vi "DIMPowerSupply.ProcCases.vi"(0 "i ref in":refnum<vi>, 1 "selector":string, 2 "Data":T1, 3 "call cluster":T2={"Object"="", "Selector"="", "CallType"=enum."synchronous", "Async Object"="", "Async Selector"="", "Data Descriptor"="", "Data"=[], "Error #"=0, "Expire"=0}, 5 "error in (no error)":errorcluster) -> (14 "i ref out":refnum<vi>, 17 "answer cluster":T2={"Object"="", "Selector"="", "CallType"=enum."synchronous", "Async Object"="", "Async Selector"="", "Data Descriptor"="", "Data"=[], "Error #"=0, "Expire"=0}, 19 "error out":errorcluster)   [LabVIEW 2014, in "DIMPowerSupply.lvlib"]
doc: "This method is called by a process from within the default case in the event loop. The methods of a class that are linked to events will be called from THIS method. Add your code here."
uses:
  DIMPowerSupply.lvlib
  CS_Core/CSSystem/CoreDefs/CoreDefs.call_type.ctl
  CS_Core/BaseProcess/BaseProcess.descriptor string definition.ctl
  CS_Core/CSSystem/CoreDefs/CoreDefs.rawDataType.ctl
  CS_Core/CSSystem/CoreLib/CoreLib.byte array 2 double.vi
  CS_Core/CSSystem/CoreLib/CoreLib.string 2 byte array.vi
  CS_Core/CSSystem/CoreLib/CoreLib.byte array 2 int.vi
  CS_Core/BaseProcess/BaseProcess.lvlib
  CS_Core/CSSystem/CoreLib/CoreLib.lvlib
  CS_Core/CAEObj/CAEObj.lvlib
  CS_Core/CSApplicationBaseClasses/PSChannelBase/PSChannelBase.lvlib
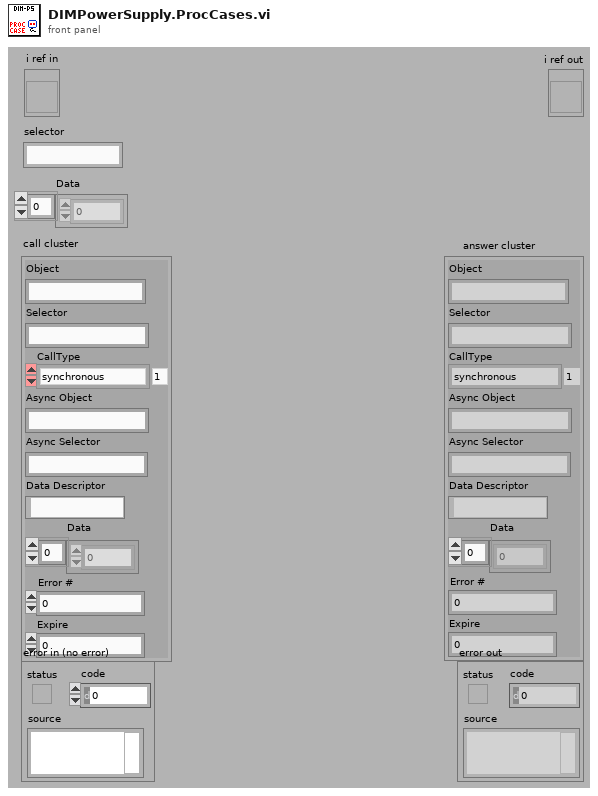
[diagram p1: front panel]
types:
  T1 = typedef "CoreDefs.rawDataType.ctl" = i8[]
  T2 = typedef "CoreDefs.call_type.ctl" = cluster{"Object":string, "Selector":string, "CallType":enum16{"simple", "synchronous", "asynchronous"}, "Async Object":string, "Async Selector":string, "Data Descriptor":T3, "Data":T1, "Error #":i32, "Expire":u32}
  T3 = typedef "BaseProcess.lvlib/BaseProcess.descriptor string definition.ctl" = string
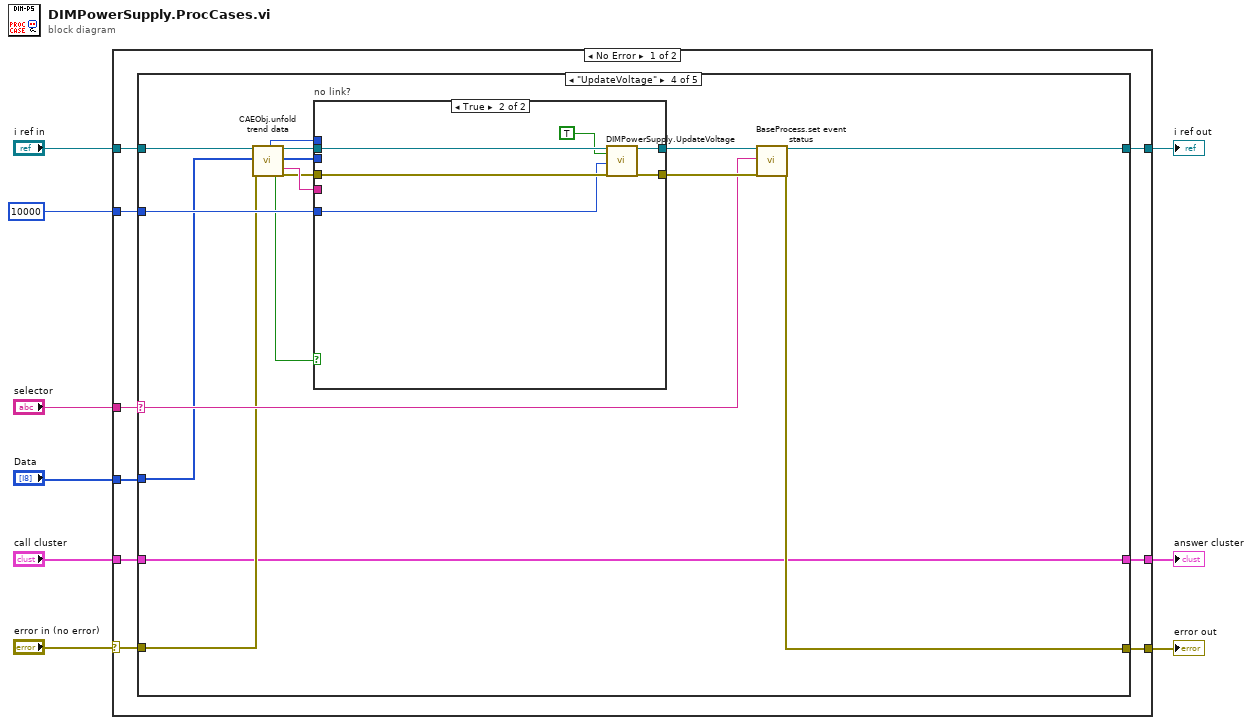
[diagram p0: block diagram]
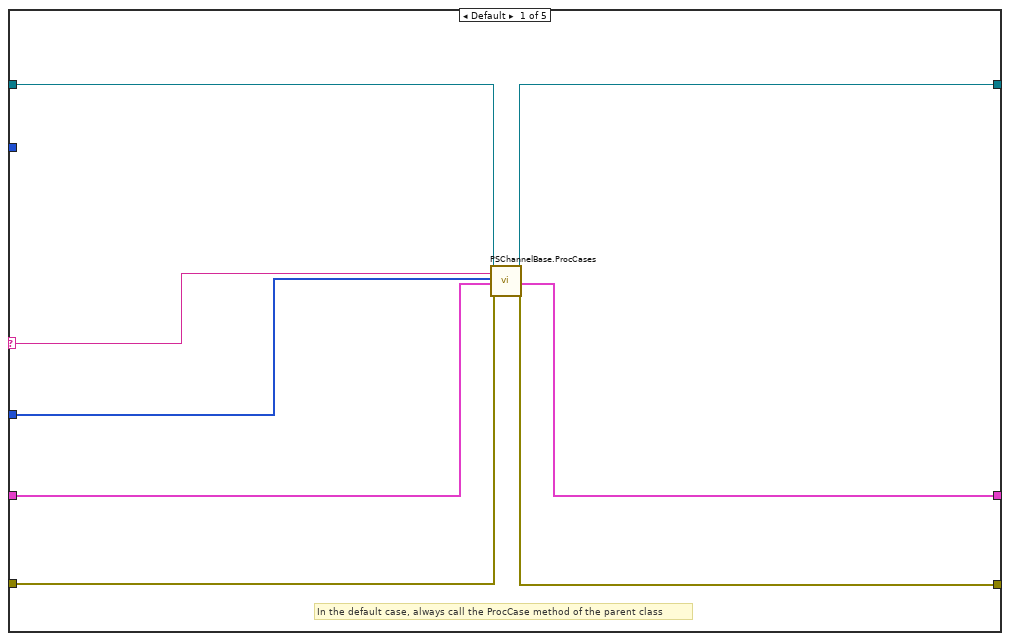
[diagram p2: hidden frame]
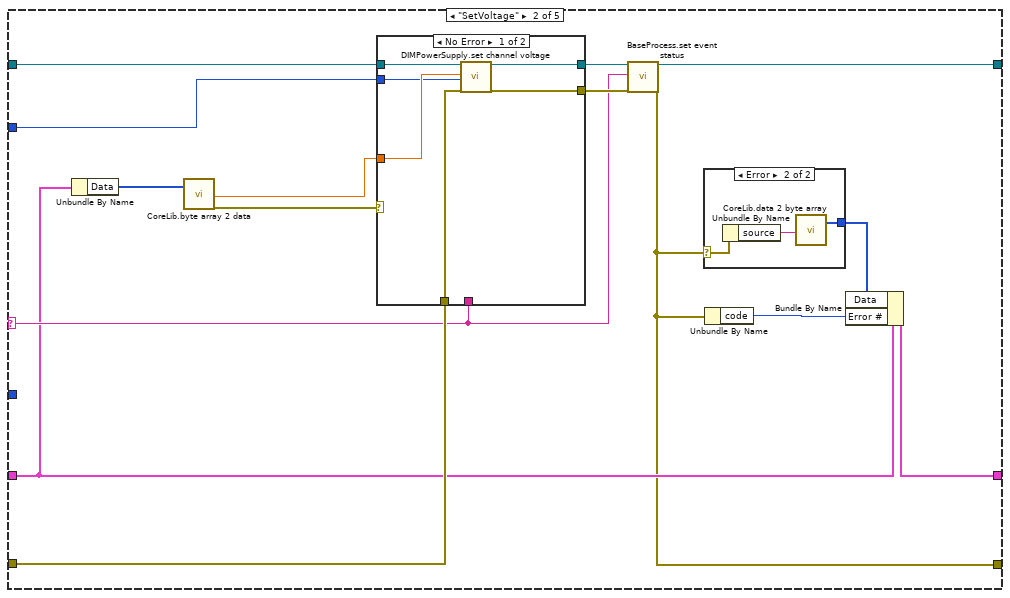
[diagram p3: hidden frame]
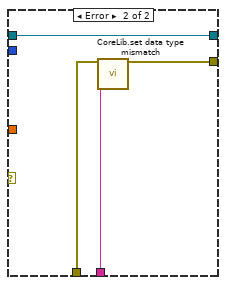
[diagram p4: hidden frame]
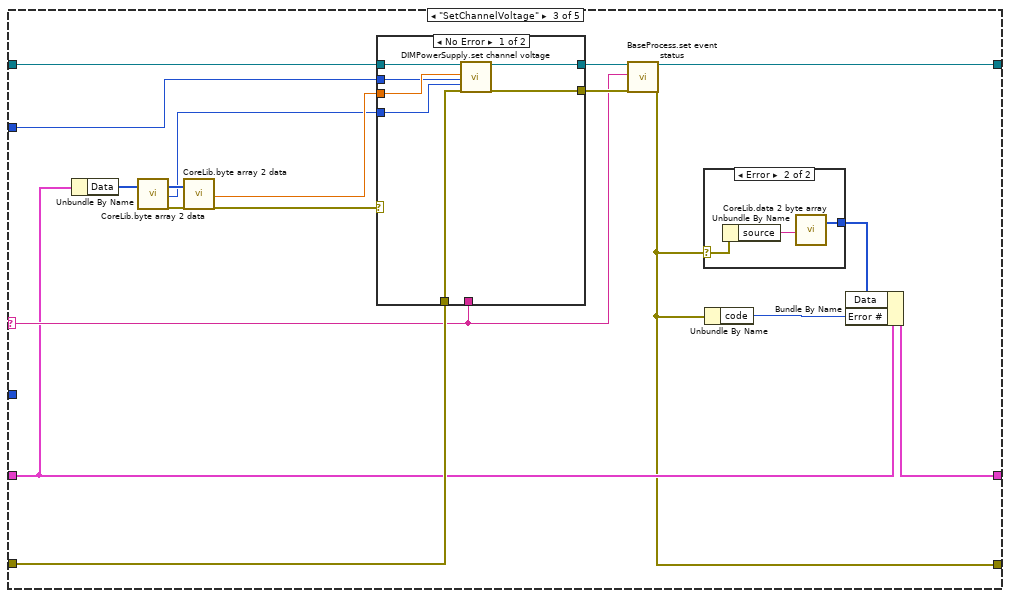
[diagram p6: hidden frame]
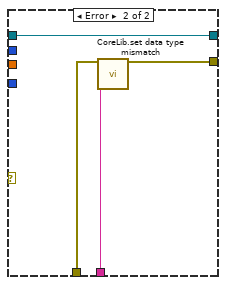
[diagram p7: hidden frame]
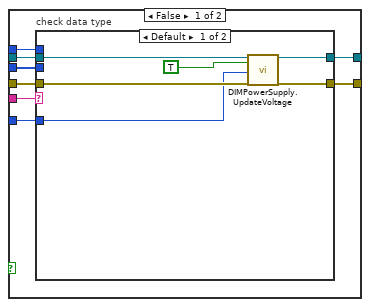
[diagram p9: hidden frame]
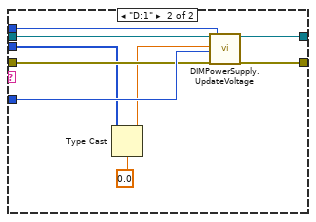
[diagram p10: hidden frame]
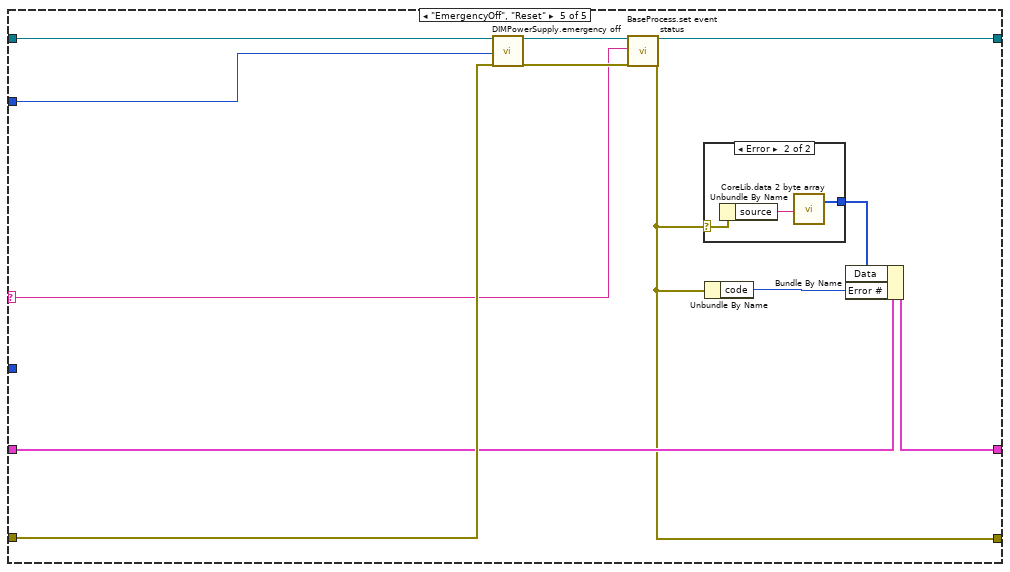
[diagram p11: hidden frame]
diagram:
  n1 = case shown="No Error" "error in (no error)" {
    selector: "error in (no error)" -> [w10 w147]
    tunnel: "selector" -> [w18 _]
    tunnel: [w17 w148] -> w8
    tunnel: "Data" -> [w16 _]
    tunnel: "call cluster" -> [w15 w148]
    tunnel: "i ref in" -> [w14 w149]
    tunnel: [w13 w149] -> w4
    tunnel: [w12 w147] -> w3
    tunnel: 10000 ("ms timeout (100)") -> [w11 _]
    frame No Error {
      n2 = case shown="\"UpdateVoltage\"" w18 {
        selector: w18 -> [w20 w35 w66 w100 w137]
        tunnel: w16 -> [w21 _ _ w96 _]
        tunnel: w14 -> [w19 w37 w68 w95 w139]
        tunnel: [w26 w30 w61 w97 w132] -> w13
        tunnel: w15 -> [w22 w33 w64 w88 w135]
        tunnel: [w23 w32 w63 w88 w134] -> w17
        tunnel: w10 -> [w25 w36 w67 w93 w138]
        tunnel: [w24 w31 w62 w98 w133] -> w12
        tunnel: w11 -> [_ w34 w65 w99 w136]
        frame Default {
          # "In the default case, always call the ProcCase method of the parent class"
          n3 = call "PSChannelBase.ProcCases.vi"("i ref in"=w19, "selector"=w20, "Data"=w21, "call cluster"=w22, "error in (no error)"=w25) -> ("i ref out"=w26:refnum<vi>, "answer cluster"=w23:T2, "error out"=w24:errorcluster)  [unwired: 12 in]
        }
        frame "SetVoltage" {
          n4 = Unbundle By Name(w33) -> ("Data"=w29:T1)
          n5 = call-poly "CoreLib.byte array 2 data.vi"("byteArray"=w29) -> ("d64"=w27:dbl, "error out"=w28:errorcluster)  [unwired: 16 in, 1 out]
          n6 = case shown="No Error" w28 {
            tunnel: [w47 w50] -> w40
            tunnel: [w46 w51] -> w41
            tunnel: w27 -> [w45 _]
            tunnel: w37 -> [w44 w50]
            tunnel: w36 -> [w43 w49]
            tunnel: w35 -> [_ w48]
            tunnel: w34 -> [w42 _]
            frame No Error {
              n7 = call "DIMPowerSupply.set channel voltage.vi"("i ref in"=w44, "Voltage"=w45, "ms timeout (10000)"=w42, "error in (no error)"=w43) -> ("i ref out"=w47:refnum<vi>, "error out"=w46:errorcluster)  [unwired: 13 in, 1 out]
            }
            frame Error {
              n8 = call "CoreLib.set data type mismatch.vi"("error in (no error)"=w49, "error source"=w48) -> ("error out"=w51:errorcluster)  [unwired: 17 in]
            }
          }
          n9 = call "BaseProcess.set event status.vi"("i ref in"=w40, "EventStatus"=w35, "error in (no error)"=w41) -> ("i ref out"=w30:refnum<vi>, "error out"=w31:errorcluster)  [unwired: 14 in, 1 out]
          n10 = case shown="Error" w31 {
            selector: w31 -> [_ w54]
            tunnel: [_ w52] -> w39
            frame No Error {
            }
            frame Error {
              n11 = Unbundle By Name(w54) -> ("source"=w53:string)
              n12 = call-poly "CoreLib.data 2 byte array.vi"("string"=w53) -> ("byteArray out"=w52:T1)  [unwired: 18 in]
            }
          }
          n13 = Unbundle By Name(w31) -> ("code"=w38:i32)
          n14 = Bundle By Name(cluster=w33, "Data"=w39, "Error #"=w38) -> (w32:T2)
        }
        frame "SetChannelVoltage" {
          n15 = Unbundle By Name(w64) -> ("Data"=w56:T1)
          n16 = call-poly "CoreLib.byte array 2 data.vi"("byteArray"=w56) -> ("byteArray out"=w58:T1, "i32"=w55:i32, "error out"=w57:errorcluster)  [unwired: 16 in]
          n17 = call-poly "CoreLib.byte array 2 data.vi"("byteArray"=w58, "error in (no error)"=w57) -> ("d64"=w59:dbl, "error out"=w60:errorcluster)  [unwired: 15 in, 1 out]
          n18 = case shown="No Error" w60 {
            tunnel: [w79 w82] -> w71
            tunnel: [w78 w83] -> w72
            tunnel: w59 -> [w77 _]
            tunnel: w68 -> [w76 w82]
            tunnel: w67 -> [w75 w81]
            tunnel: w66 -> [_ w80]
            tunnel: w65 -> [w74 _]
            tunnel: w55 -> [w73 _]
            frame No Error {
              n19 = call "DIMPowerSupply.set channel voltage.vi"("i ref in"=w76, "Voltage"=w77, "ms timeout (10000)"=w74, "channel"=w73, "error in (no error)"=w75) -> ("i ref out"=w79:refnum<vi>, "error out"=w78:errorcluster)  [unwired: 12 in, 1 out]
            }
            frame Error {
              n20 = call "CoreLib.set data type mismatch.vi"("error in (no error)"=w81, "error source"=w80) -> ("error out"=w83:errorcluster)  [unwired: 17 in]
            }
          }
          n21 = call "BaseProcess.set event status.vi"("i ref in"=w71, "EventStatus"=w66, "error in (no error)"=w72) -> ("i ref out"=w61:refnum<vi>, "error out"=w62:errorcluster)  [unwired: 14 in, 1 out]
          n22 = case shown="Error" w62 {
            selector: w62 -> [_ w86]
            tunnel: [_ w84] -> w70
            frame No Error {
            }
            frame Error {
              n23 = Unbundle By Name(w86) -> ("source"=w85:string)
              n24 = call-poly "CoreLib.data 2 byte array.vi"("string"=w85) -> ("byteArray out"=w84:T1)  [unwired: 18 in]
            }
          }
          n25 = Unbundle By Name(w62) -> ("code"=w69:i32)
          n26 = Bundle By Name(cluster=w64, "Data"=w70, "Error #"=w69) -> (w63:T2)
        }
        frame "UpdateVoltage" {
          n27 = call "CAEObj.unfold trend data.vi"("i ref in"=w95, "raw trend data"=w96, "error in (no error)"=w93) -> ("quality"=w87:i32, "no link"=w92:bool, "i ref out"=w94:refnum<vi>, "data"=w89:i8[], "typeDescriptor"=w91:string, "error out"=w90:errorcluster)  [unwired: 8 in, 3 out]
          n28 = case "no link?" shown="True" w92 {
            tunnel: [w110 w131] -> w101
            tunnel: [w109 w130] -> w102
            tunnel: w89 -> [w108 _]
            tunnel: w94 -> [w107 w129]
            tunnel: w99 -> [w106 w127]
            tunnel: w91 -> [w105 _]
            tunnel: w90 -> [w104 w128]
            tunnel: w87 -> [w103 _]
            frame False {
              n29 = case "check data type" shown="Default" w105 {
                tunnel: [w113 w125] -> w110
                tunnel: [w112 w124] -> w109
                tunnel: w108 -> [_ w120]
                tunnel: w107 -> [w115 w123]
                tunnel: w106 -> [w111 w122]
                tunnel: w104 -> [w114 w121]
                tunnel: w103 -> [_ w117]
                frame Default {
                  n30 = call "DIMPowerSupply.UpdateVoltage.vi"("i ref in"=w115, "badValue"=TRUE, "ms timeout (10000)"=w111, "error in (no error)"=w114) -> ("i ref out"=w113:refnum<vi>, "error out"=w112:errorcluster)  [unwired: 13 in, 1 out]
                }
                frame "D:1" {
                  n31 = Type Cast(type=0.0, x=w120) -> (*(type *) &x=w119:dbl)
                  n32 = call "DIMPowerSupply.UpdateVoltage.vi"("i ref in"=w123, "moduleValue"=w119, "ms timeout (10000)"=w122, "error in (no error)"=w121, "voltageQuality"=w117) -> ("i ref out"=w125:refnum<vi>, "error out"=w124:errorcluster)  [unwired: 12 in, 1 out]
                }
              }
            }
            frame True {
              n33 = call "DIMPowerSupply.UpdateVoltage.vi"("i ref in"=w129, "badValue"=TRUE, "ms timeout (10000)"=w127, "error in (no error)"=w128) -> ("i ref out"=w131:refnum<vi>, "error out"=w130:errorcluster)  [unwired: 13 in, 1 out]
            }
          }
          n34 = call "BaseProcess.set event status.vi"("i ref in"=w101, "EventStatus"=w100, "error in (no error)"=w102) -> ("i ref out"=w97:refnum<vi>, "error out"=w98:errorcluster)  [unwired: 14 in, 1 out]
        }
        frame "EmergencyOff", "Reset" {
          n35 = call "DIMPowerSupply.emergency off.vi"("i ref in"=w139, "ms timeout (10000)"=w136, "error in (no error)"=w138) -> ("i ref out"=w142:refnum<vi>, "error out"=w143:errorcluster)  [unwired: 14 in, 1 out]
          n36 = call "BaseProcess.set event status.vi"("i ref in"=w142, "EventStatus"=w137, "error in (no error)"=w143) -> ("i ref out"=w132:refnum<vi>, "error out"=w133:errorcluster)  [unwired: 14 in, 1 out]
          n37 = case shown="Error" w133 {
            selector: w133 -> [_ w146]
            tunnel: [_ w145] -> w141
            frame No Error {
            }
            frame Error {
              n38 = Unbundle By Name(w146) -> ("source"=w144:string)
              n39 = call-poly "CoreLib.data 2 byte array.vi"("string"=w144) -> ("byteArray out"=w145:T1)  [unwired: 18 in]
            }
          }
          n40 = Unbundle By Name(w133) -> ("code"=w140:i32)
          n41 = Bundle By Name(cluster=w135, "Data"=w141, "Error #"=w140) -> (w134:T2)
        }
      }
    }
    frame Error {
    }
  }
  "answer cluster" <- w8
  "i ref out" <- w4
  "error out" <- w3
